vi "Write Database.vi"(8 "error in (no error)":errorcluster, 10 "reference":T1, 11 "AcquistionObject in":refnum<class "AcquistionObject.lvclass">) -> (0 "error out":errorcluster, 3 "AcquistionObject out":refnum<class "AcquistionObject.lvclass">)   [LabVIEW 2014, in "AcquisitionCoreObjects.lvlib" / "AcquistionObject.lvclass"]
uses:
  AcquistionObject.lvclass
  <vilib>/addons/database/Connection.llb/Conn ObjectReference.ctl
  AcquistionObject.lvclass/AcquistionObject.ctl
  <vilib>/addons/database/NI_Database_API.lvlib
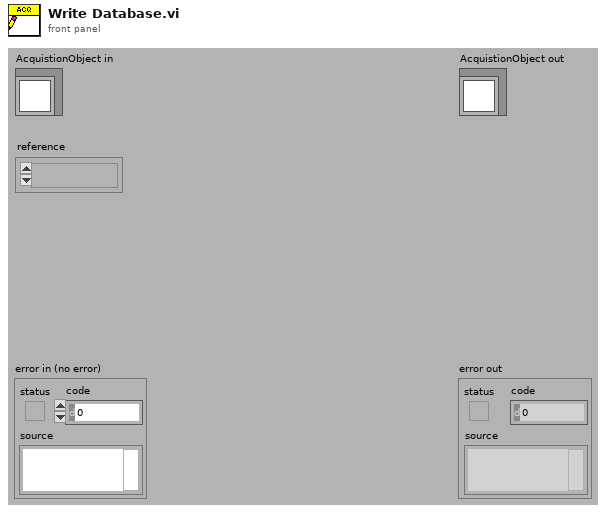
[diagram p1: front panel]
types:
  T1 = typedef "NI_Database_API.lvlib/Conn ObjectReference.ctl" = refnum<k1>
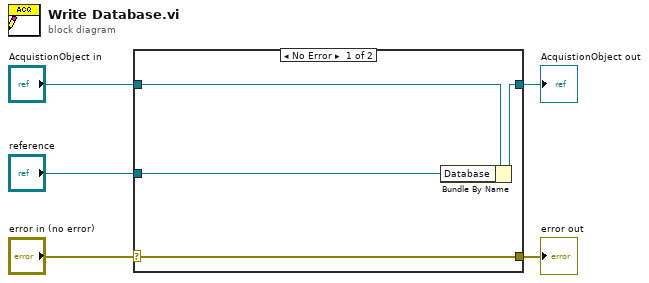
[diagram p0: block diagram]
diagram:
  n1 = case shown="No Error" "error in (no error)" {
    selector: "error in (no error)" -> [w9 w10]
    tunnel: [w9 w10] -> w4
    tunnel: [w7 w11] -> w2
    tunnel: "AcquistionObject in" -> [w8 w11]
    tunnel: "reference" -> [w6 _]
    frame No Error {
      n2 = Bundle By Name(cluster=w8, "Database"=w6) -> (w7:refnum<class "AcquistionObject.lvclass">)
    }
    frame Error {
    }
  }
  "error out" <- w4
  "AcquistionObject out" <- w2
